vi "Initialize.vi"(8 "error in (no error)":errorcluster, 11 "Channel in":refnum<class "Channel.lvclass">) -> (0 "error out":errorcluster, 3 "Channel out":refnum<class "Channel.lvclass">)   [LabVIEW 2018, in "Channel.lvclass"]
uses:
  Channel.lvclass
  Channel.lvclass/Channel.ctl
  Interface/Interface.lvclass
  StateMachine/State Machine.lvclass
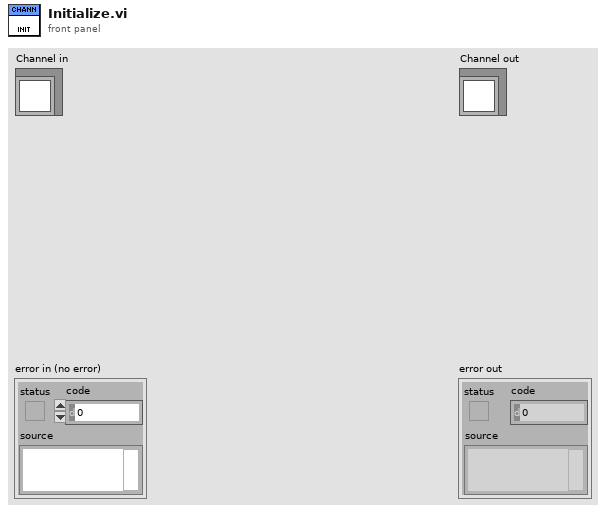
[diagram p1: front panel]
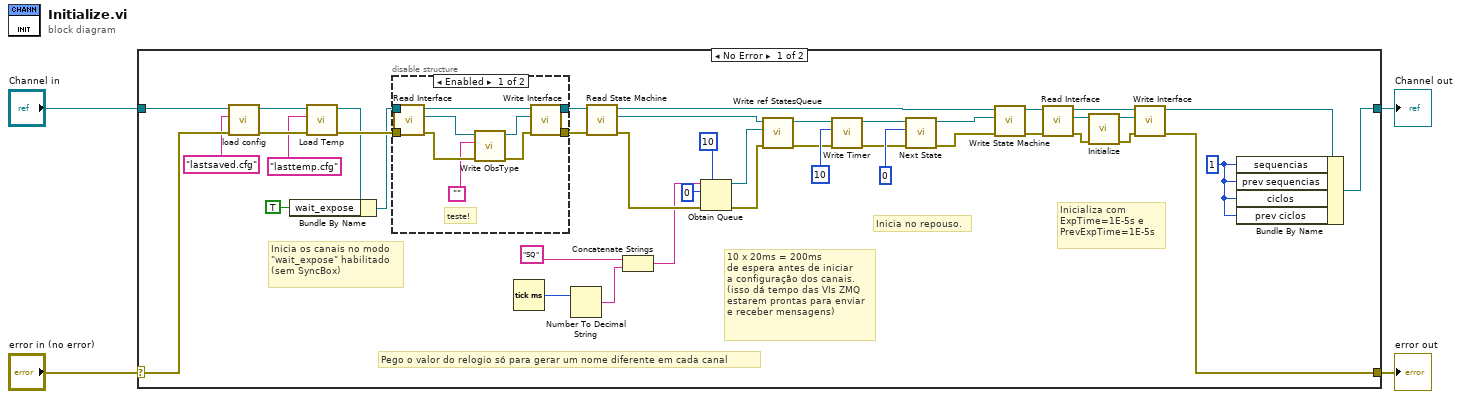
[diagram p0: block diagram]
diagram:
  n1 = case shown="No Error" "error in (no error)" {
    selector: "error in (no error)" -> [w41 w60]
    tunnel: [w10 w60] -> w3
    tunnel: [w6 w59] -> w1
    tunnel: "Channel in" -> [w42 w59]
    frame No Error {
      w5 = u32 1 ("sequencias")
      # "Inicializa com\nExpTime=1E-5s e\nPrevExpTime=1E-5s"
      # "Pego o valor do relogio só para gerar um nome diferente em cada canal"
      # "Inicia no repouso."
      # "10 x 20ms = 200ms\nde espera antes de iniciar \na configuração dos canais.\n(isso dá tempo das VIs ZMQ\nestarem prontas para enviar\ne receber mensagens)"
      # "Inicia os canais no modo\n\"wait_expose\" habilitado\n(sem SyncBox)"
      n2 = call-dynamic "load config.vi"("error in (no error)"=w41, "cfg file name"="lastsaved.cfg", "Channel in"=w42) -> ("error out"=w36:errorcluster, "Channel out"=w37:refnum<class "Channel.lvclass">)  [unwired: 7 in]
      n3 = call-dynamic "Load Temp.vi"("error in (no error)"=w36, "temp file name"="lasttemp.cfg", "Channel in"=w37) -> ("error out"=w35:errorcluster, "Channel out"=w33:refnum<class "Channel.lvclass">)  [unwired: 7 in]
      n4 = Bundle By Name(cluster=w33, "wait_expose"=TRUE) -> (w32:refnum<class "Channel.lvclass">)
      n5 = disable-structure shown="Enabled" {
        disable-tunnel: w32 -> [w56 w58]
        disable-tunnel: [w54 w58] -> w39
        disable-tunnel: w35 -> [w51 w57]
        disable-tunnel: [w48 w57] -> w38
        frame Enabled {
          # "teste!"
          n6 = call-dynamic "Read Interface.vi"("error in (no error)"=w51, "Channel in"=w56) -> ("error out"=w50:errorcluster, "Interface.lvclass"=w53:refnum<class "Interface.lvclass">, "Channel out"=w55:refnum<class "Channel.lvclass">)  [unwired: 7 in]
          n7 = call-dynamic "Write ObsType.vi"("error in (no error)"=w50, "ObsType"="" ("Acq_Status"), "Interface in"=w53) -> ("error out"=w49:errorcluster, "Interface out"=w52:refnum<class "Interface.lvclass">)  [unwired: 7 in]
          n8 = call-dynamic "Write Interface.vi"("error in (no error)"=w49, "Interface.lvclass"=w52, "Channel in"=w55) -> ("error out"=w48:errorcluster, "Channel out"=w54:refnum<class "Channel.lvclass">)  [unwired: 7 in]
        }
        frame Disabled {
        }
      }
      n9 = Tick Count (ms)() -> (millisecond timer value=w19:u32)
      n10 = Number To Decimal String(number=w19) -> (decimal integer string=w17:string)  [unwired: 1 in]
      n11 = call-dynamic "Read State Machine.vi"("error in (no error)"=w38, "Device in"=w39) -> ("error out"=w26:errorcluster, "State Machine.lvclass"=w25:refnum<class "State Machine.lvclass">, "Device out"=w44:refnum<class "Channel.lvclass">)  [unwired: 7 in]
      n12 = Concatenate Strings("SQ" ("name (unnamed)"), w17) -> (w16:string)
      n13 = Obtain Queue(max queue size (-1, unlimited)=10, name (unnamed)=w16, element data type=u32 0 ("Timer"), error in (no error)=w26) -> (queue out=w23:refnum<queue>, error out=w22:errorcluster)  [unwired: 1 in, 1 out]
      n14 = call-dynamic "Write ref StatesQueue.vi"("error in (no error)"=w22, "ref StatesQueue"=w23, "State Machine in"=w25) -> ("error out"=w21:errorcluster, "State Machine out"=w24:refnum<class "State Machine.lvclass">)  [unwired: 7 in]
      n15 = call-dynamic "Write Timer.vi"("error in (no error)"=w21, "Timer"=u32 10, "State Machine in"=w24) -> ("error out"=w28:errorcluster, "State Machine out"=w29:refnum<class "State Machine.lvclass">)  [unwired: 7 in]
      n16 = call "Next State.vi"("error in (no error)"=w28, "New_State"=0, "State Machine in"=w29) -> ("error out"=w45:errorcluster, "State Machine out"=w46:refnum<class "State Machine.lvclass">)  [unwired: 7 in]
      n17 = call-dynamic "Write State Machine.vi"("error in (no error)"=w45, "State Machine.lvclass"=w46, "Device in"=w44) -> ("error out"=w13:errorcluster, "Device out"=w15:refnum<class "Channel.lvclass">)  [unwired: 7 in]
      n18 = call-dynamic "Read Interface.vi"("error in (no error)"=w13, "Channel in"=w15) -> ("error out"=w12:errorcluster, "Interface.lvclass"=w9:refnum<class "Interface.lvclass">, "Channel out"=w14:refnum<class "Channel.lvclass">)  [unwired: 7 in]
      n19 = call-dynamic "Initialize.vi"("error in (no error)"=w12, "Interface in"=w9) -> ("error out"=w11:errorcluster, "Interface out"=w8:refnum<class "Interface.lvclass">)  [unwired: 8 in]
      n20 = call-dynamic "Write Interface.vi"("error in (no error)"=w11, "Interface.lvclass"=w8, "Channel in"=w14) -> ("error out"=w10:errorcluster, "Channel out"=w7:refnum<class "Channel.lvclass">)  [unwired: 7 in]
      n21 = Bundle By Name(cluster=w7, "sequencias"=w5, "prev sequencias"=w5, "ciclos"=w5, "prev ciclos"=w5) -> (w6:refnum<class "Channel.lvclass">)
    }
    frame Error {
    }
  }
  "error out" <- w3
  "Channel out" <- w1
